vi "optimise.vi"(8 "error in (no error)":errorcluster, 11 "DL090216RangeOffsetImageProcessor in":refnum<class "ImageProcessorDL090216RangeOffset.lvclass">) -> (0 "error out":errorcluster, 3 "DL090216RangeOffsetImageProcessor out":refnum<class "ImageProcessorDL090216RangeOffset.lvclass">)   [LabVIEW 2010, in "ImageProcessorDL090216RangeOffset.lvclass"]
uses:
  ImageProcessorDL090216RangeOffset.lvclass
  ImageProcessorDL090216RangeOffset.lvclass/ImageProcessorDL090216RangeOffset.ctl
  common/clusters/range_offset_cluster.ctl
  common/classes/Image/Image/Image.lvclass
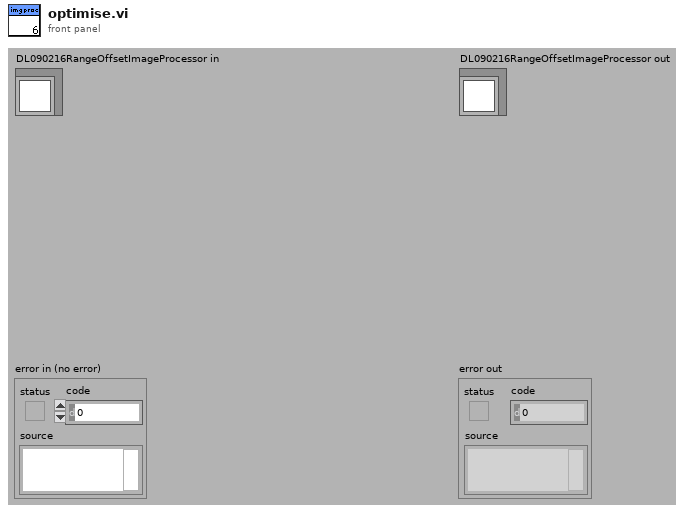
[diagram p1: front panel]
types:
  T1 = typedef "range_offset_cluster.ctl" = cluster{"range":dbl, "offset":dbl}
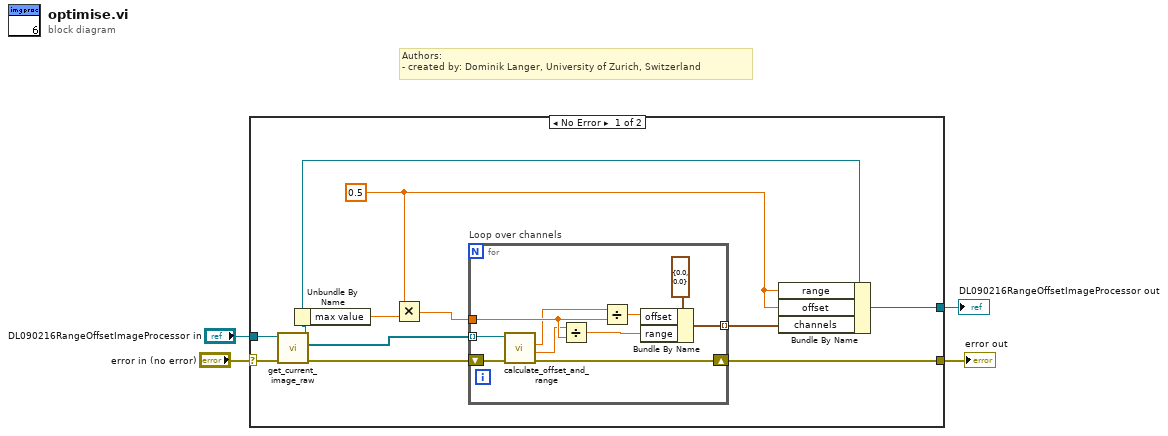
[diagram p0: block diagram]
diagram:
  # "Authors: \n- created by: Dominik Langer, University of Zurich, Switzerland"
  n1 = case shown="No Error" "error in (no error)" {
    selector: "error in (no error)" -> [w12 w27]
    tunnel: [w13 w27] -> w3
    tunnel: [w14 w26] -> w1
    tunnel: "DL090216RangeOffsetImageProcessor in" -> [w10 w26]
    frame No Error {
      w5 = 0.5 ("y")
      n2 = call-dynamic "get_current_image_raw.vi"("error in (no error)"=w12, "GenericImageProcessor.lvclass in"=w10) -> ("error out"=w11:errorcluster, "current image (channels)"=w8:refnum<class "Image.lvclass">[], "GenericImageProcessor.lvclass out"=w9:refnum<class "ImageProcessorDL090216RangeOffset.lvclass">)  [unwired: 7 out]
      n3 = Unbundle By Name(w9) -> ("max value"=w7:dbl)
      n4 = Multiply(x=w5, y=w7) -> (x*y=w6:dbl)
      n5 = for "Loop over channels" {
        shift-right: [w22] -> w13
        shift-left: w11 -> [w25]
        tunnel: w8 -> [w24] mode=indexing
        tunnel: w6 -> [w23]
        tunnel: [w18] -> w15 mode=indexing
        n6 = call-dynamic "calculate_offset_and_range.vi"("error in (no error)"=w25, "Image in"=w24) -> ("error out"=w22:errorcluster, "range"=w16:dbl, "offset / minimum"=w17:dbl)  [unwired: 7 out]
        n7 = Divide(x=w16, y=w23) -> (x/y=w20:dbl)
        n8 = Divide(x=w17, y=w23) -> (x/y=w19:dbl)
        n9 = Bundle By Name(cluster=T1 {"range"=0.0, "offset"=0.0} ("master"), "offset"=w19, "range"=w20) -> (w18:T1)
      }
      n10 = Bundle By Name(cluster=w9, "range"=w5, "offset"=w5, "channels"=w15) -> (w14:refnum<class "ImageProcessorDL090216RangeOffset.lvclass">)
    }
    frame Error {
    }
  }
  "error out" <- w3
  "DL090216RangeOffsetImageProcessor out" <- w1
